vi "Scrape Screenpops.vi"(8 "error in":errorcluster, 11 "SR number list in":i32[](array[numeric])) -> (0 "error out":errorcluster, 3 "sr clusters out":T2[](array[typedef]) {"Creation Date" format="%<%x>T"; "Last Updated" format="%<%x>T"})   [LabVIEW 2018]
uses:
  SR Cluster.ctl
  SR Status.ctl
  SR Note Cluster.ctl
  <vilib>/httpClient/LabVIEWHTTPClient.lvlib
panel:
  out "sr notes array out":T1[][](array[typedef]) {"Note Date" format="%<%x >T"}
  out "SR Note Array":T1[](array[typedef]) {"Note Date" format="%<%x >T"}
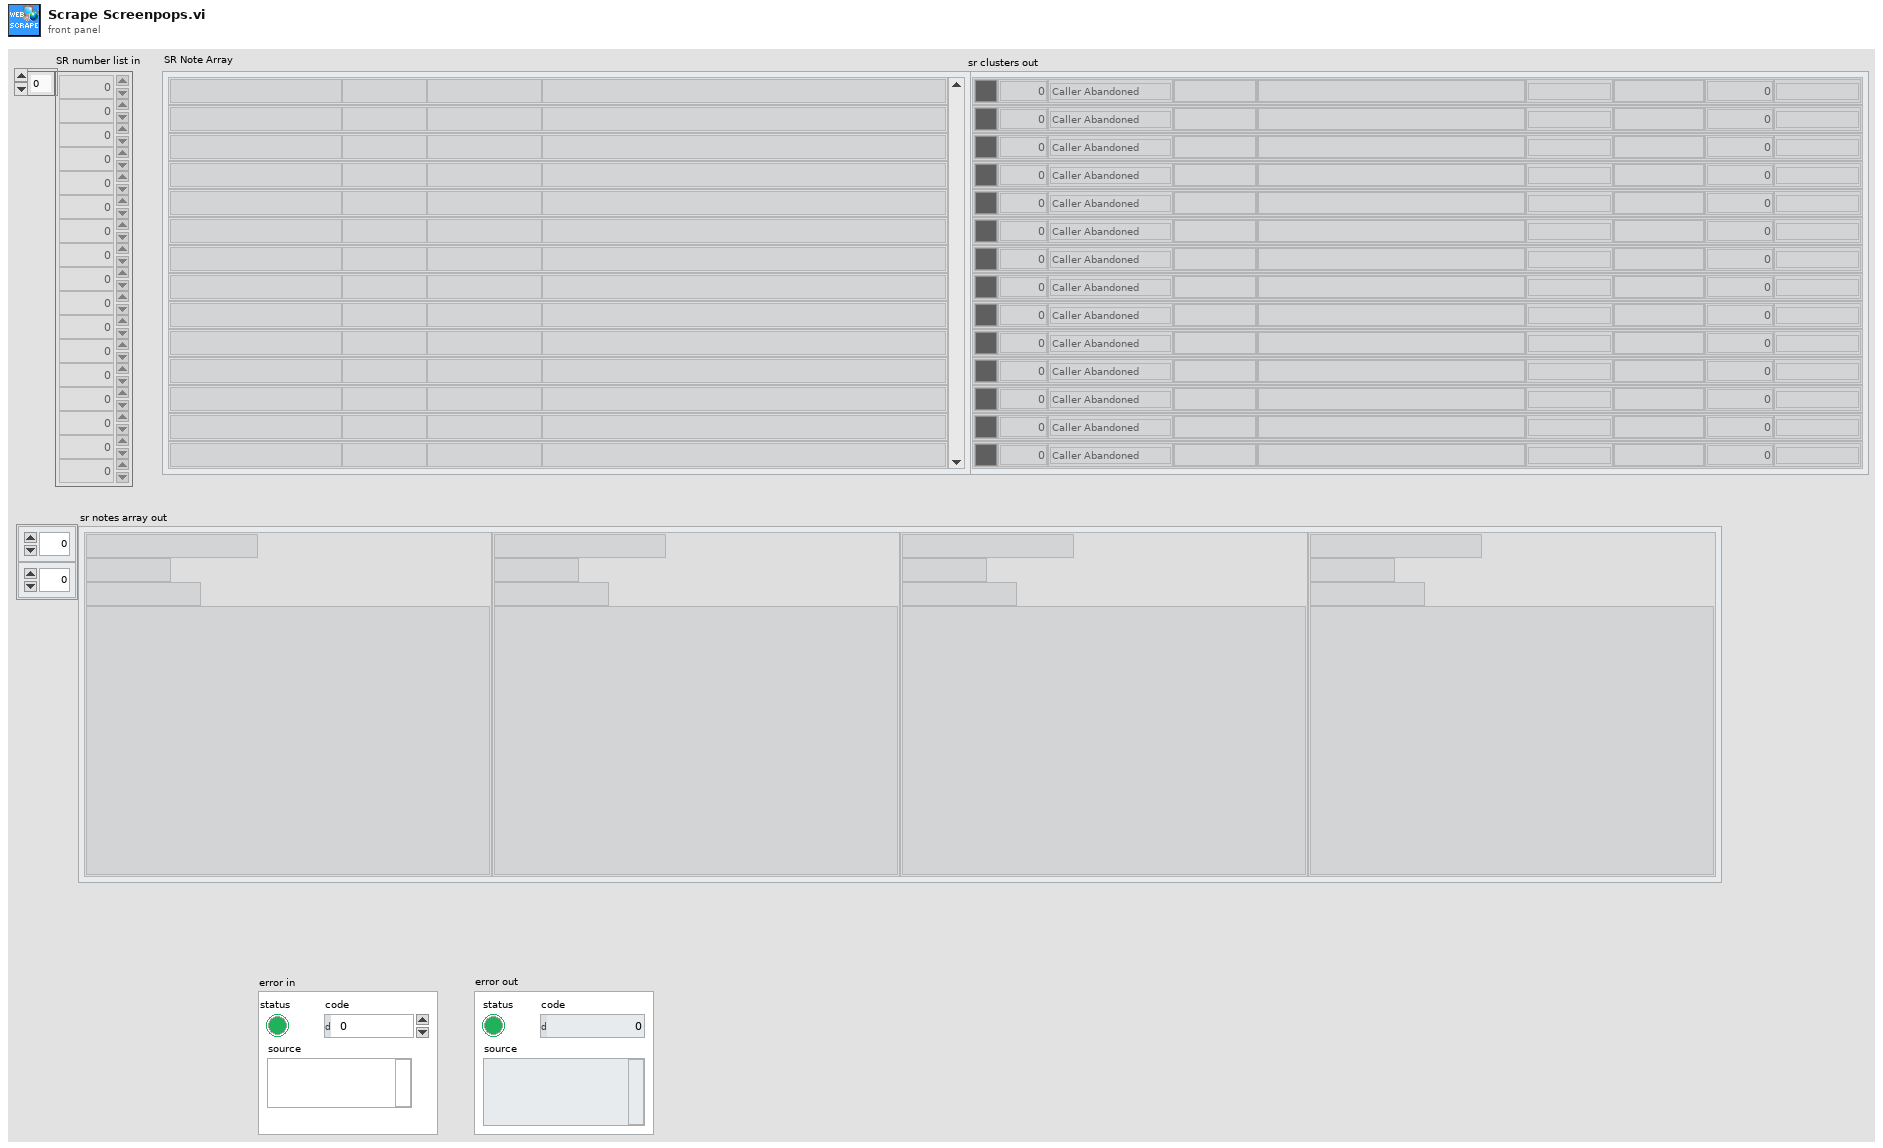
[diagram p1: front panel]
types:
  T1 = typedef "SR Note Cluster.ctl" = cluster{"Note Type":string, "Note Date":timestamp, "AE":string, "Note Text":string}
  T2 = typedef "SR Cluster.ctl" = cluster{"Color":u32, "SR Number":i32, "SR Status":T3, "SR Type":string, "Summary":string, "Last Updated":timestamp, "Service Level":string, "Days Open":dbl, "Creation Date":timestamp}
  T3 = typedef "SR Status.ctl" = enum16{"Caller Abandoned", "Created in Error", "Expired", "Forum Resolved AE", "Forum Resolved Customer", "IN WORK", "IN WORK Collab with AES", "IN WORK Collab with PSE", "IN WORK Collab with SE", "IN WORK Customer Added Note", "IN WORK Escalation", "IN WORK Wait on Customer", "Open", "Potentially Resolved", "Presumed Resolved", "RMA Approved for Return", "Resolved", "Passed Off"}
  T4 = typedef "LabVIEWHTTPClient.lvlib/ClientHandle.ctl" = refnum<k1>
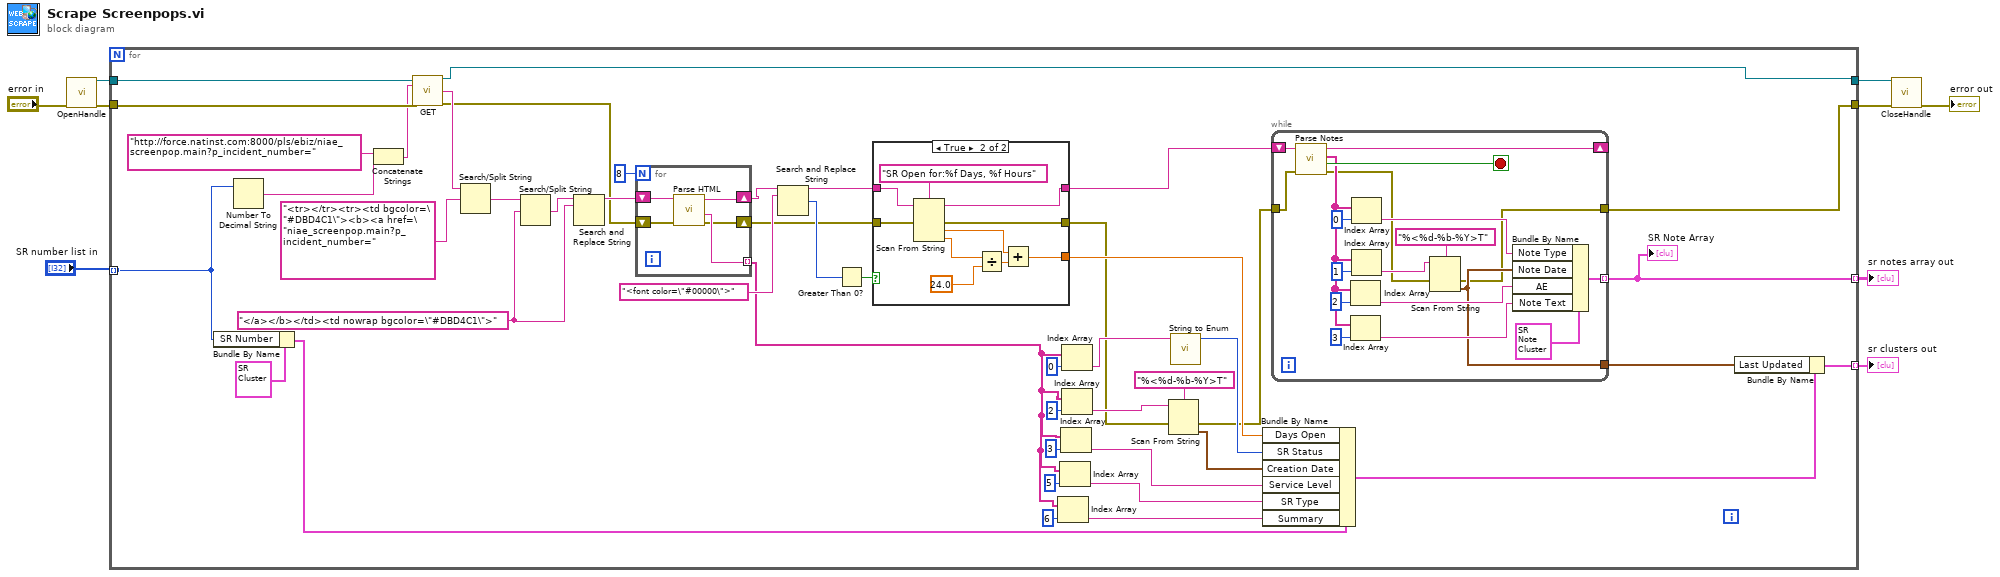
[diagram p0: block diagram]
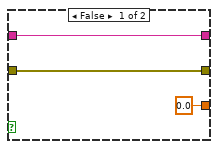
[diagram p2: hidden frame]
diagram:
  n1 = call <vilib>:"OpenHandle.vi"("error in (no error)"="error in") -> ("client handle out"=w9:T4, "error out"=w8:errorcluster)  [unwired: 13 in]
  n2 = for {
    tunnel: "SR number list in" -> [w15] mode=indexing
    tunnel: [w24] -> w5 mode=indexing
    tunnel: w8 -> [w54]
    tunnel: [w12] -> w6
    tunnel: w9 -> [w55]
    tunnel: [w14] -> w7
    tunnel: [w10] -> w1 mode=indexing
    w47 = "</a></b></td><td nowrap bgcolor=\"#DBD4C1\">" ("search string/char (-)")
    n3 = Bundle By Name(cluster=T2 {"Color"=0, "SR Number"=0, "SR Status"=enum."Caller Abandoned", "SR Type"="", "Summary"="", "Last Updated"=timestamp(0 s since 1904-01-01), "Service Level"="", "Days Open"=0.0, "Creation Date"=timestamp(0 s since 1904-01-01)} ("SR Cluster"), "SR Number"=w15) -> (w29:T2)
    n4 = Number To Decimal String(number=w15) -> (decimal integer string=w53:string)  [unwired: 1 in]
    n5 = Concatenate Strings("http://force.natinst.com:8000/pls/ebiz/niae_screenpop.main?p_incident_number=" ("string"), w53) -> (w52:string)
    n6 = call <vilib>:"GET.vi"("client handle"=w55, "url"=w52, "error in (no error)"=w54) -> ("client handle out"=w14:T4, "body"=w51:string, "error out"=w18:errorcluster)  [unwired: 9 in, 1 out]
    n7 = Search/Split String(string=w51, search string/char (-)="<tr></tr><tr><td bgcolor=\"#DBD4C1\"><b><a href=\"niae_screenpop.main?p_incident_number=") -> (match + rest of string=w44:string)  [unwired: 1 in, 2 out]
    n8 = Search/Split String(string=w44, search string/char (-)=w47) -> (match + rest of string=w46:string)  [unwired: 1 in, 2 out]
    n9 = Search and Replace String(input string=w46, search string=w47) -> (result string=w48:string)  [unwired: 6 in, 3 out]
    n10 = for {
      N: 8 -> [_]
      shift-right: [w91] -> w22
      shift-left: w48 -> [w92]
      tunnel: [w90] -> w33 mode=indexing
      shift-right: [w89] -> w17
      shift-left: w18 -> [w88]
      n11 = call "Parse HTML.vi"("error in"=w88, "result string in"=w92) -> ("error out"=w89:errorcluster, "data"=w90:string, "result string out"=w91:string)  [unwired: 7 in]
    }
    n12 = Search and Replace String(input string=w22, search string="<font color=\"#00000\">") -> (result string=w20:string, number of replacements=w21:i32)  [unwired: 6 in, 2 out]
    n13 = Greater Than 0?(x=w21) -> (x > 0?=w23:bool)
    n14 = case shown="True" w23 {
      tunnel: w20 -> [w77 w87]
      tunnel: [w77 w83] -> w43
      tunnel: [0.0 w82] -> w39
      tunnel: w17 -> [w75 w79]
      tunnel: [w75 w78] -> w19
      frame False {
      }
      frame True {
        n15 = Scan From String(format string="SR Open for:%f Days, %f Hours", input string=w87, error in=w79) -> (remaining string=w83:string, error out=w78:errorcluster, output 1=w80:dbl, output 2=w85:dbl)  [unwired: 3 in, 1 out]
        n16 = Divide(x=w85, y=24.0) -> (x/y=w81:dbl)
        n17 = Add(x=w80, y=w81) -> (x+y=w82:dbl)
      }
    }
    n18 = Index Array(array=w33, index=6) -> (element=w30:string)
    n19 = Index Array(array=w33, index=5) -> (element=w31:string)
    n20 = Index Array(array=w33, index=3) -> (element=w32:string)
    n21 = Index Array(array=w33, index=0) -> (element=w38:string)
    n22 = Index Array(array=w33, index=2) -> (element=w27:string)
    n23 = Scan From String(format string="%<%d-%b-%Y>T", input string=w27, error in=w19) -> (error out=w16:errorcluster, output 1=w26:timestamp)  [unwired: 2 in, 2 out]
    n24 = call "String to Enum.vi"("string in"=w38) -> ("enum out"=w37:T3)  [unwired: 9 in, 1 out]
    n25 = Bundle By Name(cluster=w29, "Days Open"=w39, "SR Status"=w37, "Creation Date"=w26, "Service Level"=w32, "SR Type"=w31, "Summary"=w30) -> (w25:T2)
    n26 = while {
      shift-right: [w73] -> _
      shift-left: w43 -> [w74]
      tunnel: w16 -> [w71]
      tunnel: [w56] -> w12
      tunnel: [w59] -> w10 mode=indexing
      tunnel: [w58] -> w11
      stop <- w72 stop-if-true
      n27 = call "Parse Notes.vi"("error in"=w71, "String"=w74) -> ("error out"=w57:errorcluster, "Done Reading?"=w72:bool, "sr note out"=w70:string[], "result string out"=w73:string)  [unwired: 6 in]
      n28 = Index Array(array=w70, index=2) -> (element=w63:string)
      n29 = Index Array(array=w70, index=3) -> (element=w64:string)
      n30 = Index Array(array=w70, index=0) -> (element=w61:string)
      n31 = Index Array(array=w70, index=1) -> (element=w60:string)
      n32 = Scan From String(format string="%<%d-%b-%Y>T", input string=w60, error in=w57) -> (error out=w56:errorcluster, output 1=w58:timestamp)  [unwired: 2 in, 2 out]
      n33 = Bundle By Name(cluster=T1 {"Note Type"="", "Note Date"=timestamp(0 s since 1904-01-01), "AE"="", "Note Text"=""} ("SR Note Cluster"), "Note Type"=w61, "Note Date"=w58, "AE"=w63, "Note Text"=w64) -> (w59:T1)
    }
    "SR Note Array" <- w10
    n34 = Bundle By Name(cluster=w25, "Last Updated"=w11) -> (w24:T2)
  }
  "sr clusters out" <- w5
  "sr notes array out" <- w1
  n35 = call <vilib>:"CloseHandle.vi"("client handle"=w7, "error in (no error)"=w6) -> ("error out"=→"error out":errorcluster)  [unwired: 13 in]
